vi "Configure Arbitrary Waveform.vi"(4 "EFile Name (\"\")":string, 6 "User Waveform (0)":i32, 7 "Built-in Waveform Name (\"StairDown\")":string="StairDown", 8 "error in (no error)":errorcluster, 9 "Arbitrary Waveform Type (0: Built-in)":u16(ring) items=["Built-in", "User Waveform", "Edit Memory", "EFile"], 10 "Channel (1: Channel 1)":u16(ring)=1 items=["Channel 1"=1, "Channel 2"=2], 11 "VISA resource name":refnum<visa-resource-name>) -> (0 "error out":errorcluster, 3 "VISA resource name out":refnum<visa-resource-name>)   [LabVIEW 2016, in "Tektronix AFG 1000 Series.lvlib"]
doc: "Configures the waveform type for the arbitrary waveform generation. Use the Configure Waveform.vi to set other properties."
uses:
  Tektronix AFG 1000 Series.lvlib
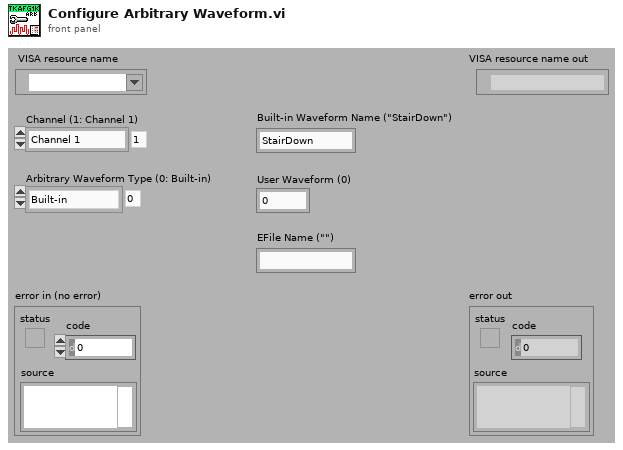
[diagram p1: front panel]
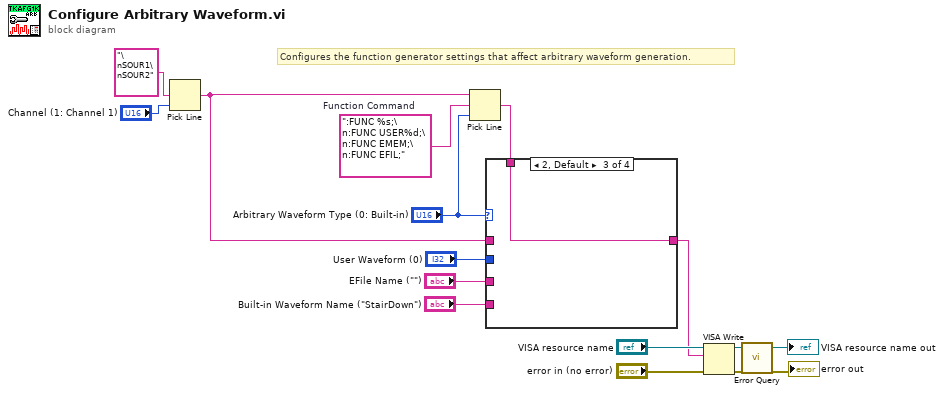
[diagram p0: block diagram]
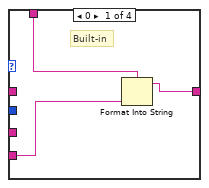
[diagram p2: hidden frame]
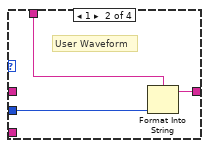
[diagram p3: hidden frame]
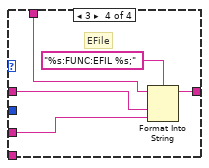
[diagram p4: hidden frame]
diagram:
  w7 = ":FUNC %s;\n:FUNC USER%d;\n:FUNC EMEM;\n:FUNC EFIL;"  # Function Command
  # "Configures the function generator settings that affect arbitrary waveform generation."
  n1 = Pick Line(multi-line string="\nSOUR1\nSOUR2" ("string (\"\")"), line index="Channel (1: Channel 1)") -> (output string=w4:string)  [unwired: 1 in]
  n2 = Pick Line(string ("")=w4, multi-line string=w7, line index="Arbitrary Waveform Type (0: Built-in)") -> (output string=w6:string)
  n3 = case shown="2, Default" "Arbitrary Waveform Type (0: Built-in)" {
    tunnel: w6 -> [w19 w22 w23 w27]
    tunnel: [w18 w21 w23 w28] -> w1
    tunnel: w4 -> [_ _ _ w25]
    tunnel: "EFile Name (\"\")" -> [_ _ _ w24]
    tunnel: "User Waveform (0)" -> [_ w20 _ _]
    tunnel: "Built-in Waveform Name (\"StairDown\")" -> [w17 _ _ _]
    frame 0 {
      # "Built-in"
      n4 = Format Into String(format string=w19, w17) -> (resulting string=w18:string)  [unwired: 2 in, 1 out]
    }
    frame 1 {
      # "User Waveform"
      n5 = Format Into String(format string=w22, w20) -> (resulting string=w21:string)  [unwired: 2 in, 1 out]
    }
    frame 2, Default {
    }
    frame 3 {
      # "EFile"
      n6 = Format Into String(format string="%s:FUNC:EFIL %s;", initial string=w27, w25, w24) -> (resulting string=w28:string)  [unwired: 1 in, 1 out]
    }
  }
  n7 = VISA Write(VISA resource name="VISA resource name", write buffer=w1, error in (no error)="error in (no error)") -> (VISA resource name out=w14:refnum<visa-resource-name>, error out=w13:errorcluster)  [unwired: 1 out]
  n8 = call "Error Query.vi"("error in (no error)"=w13, "VISA resource name"=w14) -> ("error out"=→"error out":errorcluster, "VISA resource name out"=→"VISA resource name out":refnum<visa-resource-name>)  [unwired: 6 in, 2 out]
